vi "Encode Parameters to Words.vi"(8 "error in":errorcluster, 9 "message":T1={"name"="", "message type"="BC to RT", "endpoint Tx"={"terminal address"=0, "subaddress"=0}, "endpoint Rx"={"terminal address"=0, "subaddress"=0}, "create timestamp channel"=FALSE, "mode code"=0, "number of words"=0, "parameters"=[]}, 10 "Values":dbl[](array[numeric]), 11 "value index":i32) -> (0 "error out":errorcluster, 3 "data words":u16[](array[numeric]) format="%04x")   [LabVIEW 2023, in "Ballard MIL-STD-1553 Engine Support.lvlib" / "Implementation.lvlib" / "Tx Execution Unit.lvclass"]
uses:
  Tx Execution Unit.lvclass
  Shared/Message Definition.ctl
  Shared/Message Type.ctl
  Shared/Terminal Endpoint.ctl
  Shared/Address.ctl
  Shared/Parameter Definition.ctl
  57287a39-98a1-4235-a14c-2bf7a66eb33b.vi
  3ea03746-6f70-437b-b143-209d604836ee.vi
  57287a39-98a1-4235-a14c-2bf7a66eb33b.vi/136dcdcb-2dd3-4a4d-a796-a8f7a3f8e1ac.vi
  57287a39-98a1-4235-a14c-2bf7a66eb33b.vi/a54b505c-1216-4ef4-8378-3ceda9d188df.vi
  3ea03746-6f70-437b-b143-209d604836ee.vi/9377bb8f-44b5-4a8f-87f1-966fd5a9edcc.vi
  3ea03746-6f70-437b-b143-209d604836ee.vi/e95d9d1f-307c-44d6-9f26-c3f519a4990d.vi
  3ea03746-6f70-437b-b143-209d604836ee.vi/0c23f515-4369-4514-bc3d-4444e6b437b2.vi
  <vilib>/NI/NI VeriStand Encoding and Decoding/Get Bits Per Digit from Base.vi
  <vilib>/NI VeriStand/Custom Device Tools/Custom Device Utility Library/Custom Device Utility Library.lvlib
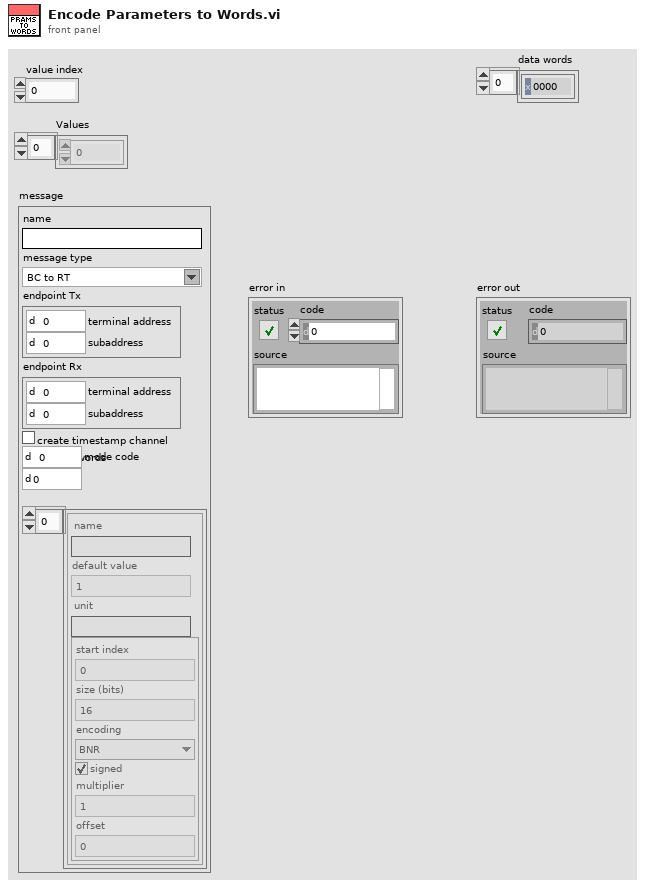
[diagram p1: front panel]
types:
  T1 = typedef "Message Definition.ctl" = cluster{"name":string, "message type":T2, "endpoint Tx":T3, "endpoint Rx":T3, "create timestamp channel":bool, "mode code":u16, "number of words":u16, "parameters":cluster{"name":string, "default value":dbl, "unit":string, "parameter definition":T5}[]}
  T2 = typedef "Message Type.ctl" = string
  T3 = typedef "Terminal Endpoint.ctl" = cluster{"terminal address":T4, "subaddress":T4}
  T4 = typedef "Address.ctl" = u16
  T5 = typedef "Parameter Definition.ctl" = cluster{"start index":i32, "size (bits)":i32, "encoding":enum16{"BNR", "BCD", "Discrete"}, "signed":bool, "multiplier":dbl, "offset":dbl}
  T6 = cluster{"name":string, "default value":dbl, "unit":string, "parameter definition":T5}[]
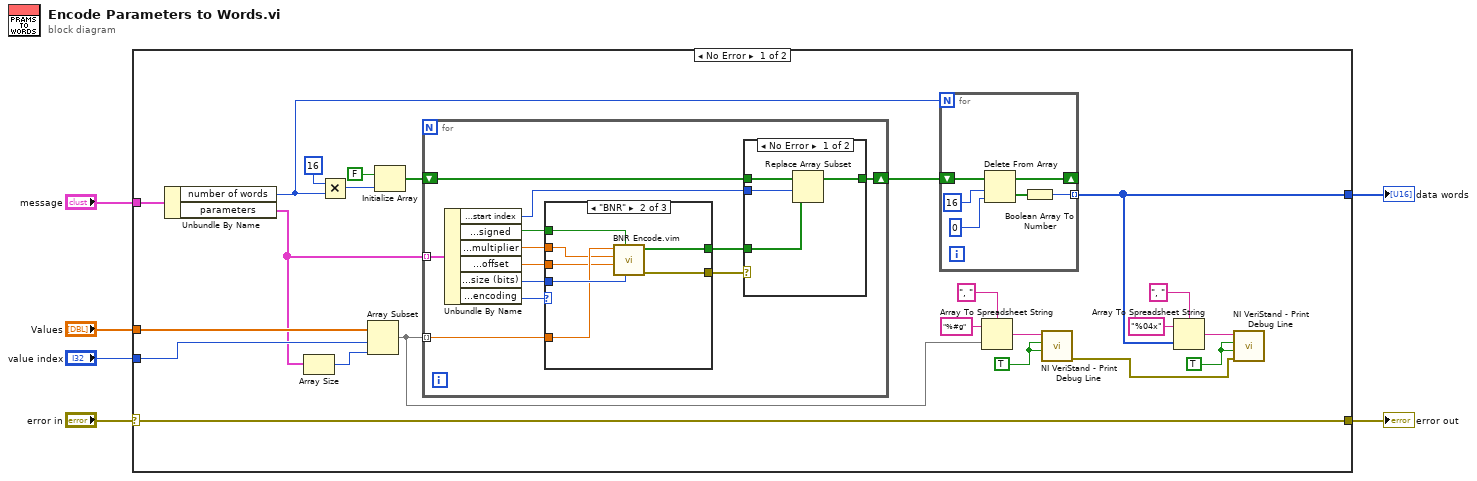
[diagram p0: block diagram]
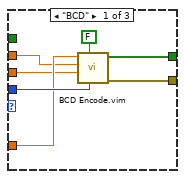
[diagram p3: hidden frame]
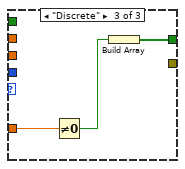
[diagram p4: hidden frame]
diagram:
  n1 = case shown="No Error" "error in" {
    selector: "error in" -> [w18 w70]
    tunnel: "message" -> [w29 _]
    tunnel: [w18 w70] -> w4
    tunnel: [w8 _] -> w3
    tunnel: "Values" -> [w22 _]
    tunnel: "value index" -> [w21 _]
    frame No Error {
      w12 = TRUE ("Append newline? (T)")
      w14 = TRUE ("Append newline? (T)")
      n2 = Unbundle By Name(w29) -> ("number of words"=w24:u16, "parameters"=w20:T6)
      n3 = Array Size(array=w20) -> (size(s)=w19:i32)
      n4 = Multiply(x=u16 16, y=w24) -> (x*y=w27:u16)
      n5 = Array Subset(array=w22, index=w21, length=w19) -> (w13:dbl[])
      n6 = Initialize Array(FALSE, w27) -> (w25:bool[])
      n7 = for {
        shift-right: [w37] -> w23
        shift-left: w25 -> [w38]
        tunnel: w20 -> [w47] mode=indexing
        tunnel: w13 -> [w46] mode=indexing
        n8 = Unbundle By Name(w47) -> ("parameter definition.start index"=w39:i32, "parameter definition.signed"=w44:bool, "parameter definition.multiplier"=w43:dbl, "parameter definition.offset"=w42:dbl, "parameter definition.size (bits)"=w41:i32, "parameter definition.encoding"=w45:enum16{"BNR", "BCD", "Discrete"})
        n9 = case shown="\"BNR\"" w45 {
          tunnel: w46 -> [w57 w63 w69]
          tunnel: w44 -> [_ w66 _]
          tunnel: w43 -> [w56 w62 _]
          tunnel: w42 -> [w55 w61 _]
          tunnel: w41 -> [w58 w64 _]
          tunnel: [w54 w65 _] -> w36
          tunnel: [w53 w60 w68] -> w40
          frame "BCD" {
            n10 = call "BCD Encode.vim"("data size (bits)"=w58, "signed"=FALSE, "scale offset"=w55, "scale multiplier"=w56, "value"=w57) -> ("error out"=w54:errorcluster, "BCD encoded value"=w53:bool[])  [unwired: 4 in, 1 out]
          }
          frame "BNR" {
            n11 = call "BNR Encode.vim"("data size (bits)"=w64, "signed"=w66, "scale offset"=w61, "scale multiplier"=w62, "value"=w63) -> ("error out"=w65:errorcluster, "BNR encoded value"=w60:bool[])  [unwired: 5 in]
          }
          frame "Discrete" {
            n12 = Not Equal To 0?(x=w69) -> (x != 0?=w67:bool)
            n13 = Build Array(w67) -> (w68:bool[])
          }
        }
        n14 = case shown="No Error" w36 {
          tunnel: w40 -> [w51 _]
          tunnel: w39 -> [w50 _]
          tunnel: w38 -> [w49 w52]
          tunnel: [w48 w52] -> w37
          frame No Error {
            n15 = Replace Array Subset(array=w49, new element=w51, index=w50) -> (w48:bool[])
          }
          frame Error {
            # "use previous value on error"
          }
        }
      }
      n16 = for {
        N: w24 -> [_]
        shift-right: [w34] -> _
        shift-left: w23 -> [w35]
        tunnel: [w30] -> w8 mode=indexing
        n17 = Delete From Array(array=w35, length=16 ("index"), index=0) -> (deleted portion=w31:bool[], array with subset deleted=w34:bool[])
        n18 = Boolean Array To Number(Boolean array=w31) -> (number=w30:u16)
      }
      n19 = Array To Spreadsheet String(delimiter (Tab)=", ", array=w13, 3:"%#g" ("format string")) -> (spreadsheet string=w15:string)
      n20 = call <vilib>:"NI VeriStand - Print Debug Line.vi"("Append newline? (T)"=w14, "Add to log file? (F)"=w14, "Message"=w15) -> ("error out"=w7:errorcluster)  [unwired: 8 in]
      n21 = Array To Spreadsheet String(delimiter (Tab)=", ", array=w8, 3:"%04x" ("format string")) -> (spreadsheet string=w11:string)
      n22 = call <vilib>:"NI VeriStand - Print Debug Line.vi"("error in (no error)"=w7, "Append newline? (T)"=w12, "Add to log file? (F)"=w12, "Message"=w11) -> ()  [unwired: 7 in, 1 out]
    }
    frame Error {
    }
  }
  "data words" <- w3
  "error out" <- w4
